vi "Get Random Monitor Edge Point.vi"(7 "Edge":enum16{"Left", "Top", "Right", "Bottom"}(ring), 10 "Monitor Bounds":T2) -> (2 "Point":T1)   [LabVIEW 2019, in "Window.lvlib"]
doc: "Get a random point on the specified edge of a given bounds rectangle, where the point is in the middle 80% of the edge."
uses:
  Window.lvlib
  <vilib>/numeric/Random Number (Range) I64.vi
  _2D/Point.ctl
  _2D/2D.lvlib
  <vilib>/Utility/miscctls.llb/LVRectTypeDef.ctl
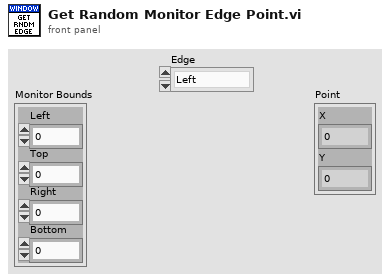
[diagram p1: front panel]
types:
  T1 = typedef "2D.lvlib/Point.ctl" = cluster{"X":i16, "Y":i16}
  T2 = typedef "LVRectTypeDef.ctl" = cluster{"Left":i16, "Top":i16, "Right":i16, "Bottom":i16}
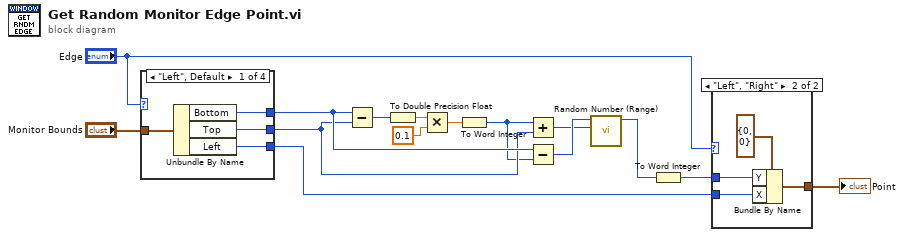
[diagram p0: block diagram]
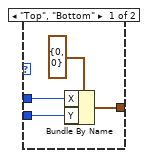
[diagram p2: hidden frame]
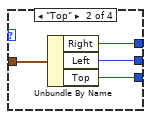
[diagram p3: hidden frame]
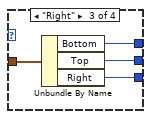
[diagram p4: hidden frame]
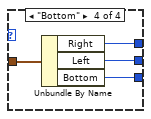
[diagram p5: hidden frame]
diagram:
  n1 = case shown="\"Left\", Default" "Edge" {
    tunnel: [w19 w23 w27 w31] -> w12
    tunnel: [w18 w22 w26 w30] -> w10
    tunnel: "Monitor Bounds" -> [w17 w21 w25 w29]
    tunnel: [w16 w20 w24 w28] -> w6
    frame "Left", Default {
      n2 = Unbundle By Name(w17) -> ("Bottom"=w19:i16, "Top"=w18:i16, "Left"=w16:i16)
    }
    frame "Top" {
      n3 = Unbundle By Name(w21) -> ("Right"=w23:i16, "Left"=w22:i16, "Top"=w20:i16)
    }
    frame "Right" {
      n4 = Unbundle By Name(w25) -> ("Bottom"=w27:i16, "Top"=w26:i16, "Right"=w24:i16)
    }
    frame "Bottom" {
      n5 = Unbundle By Name(w29) -> ("Right"=w31:i16, "Left"=w30:i16, "Bottom"=w28:i16)
    }
  }
  n6 = Subtract(x=w12, y=w10) -> (x-y=w15:i16)
  n7 = To Double Precision Float(number=w15) -> (double precision float=w14:dbl)
  n8 = Multiply(x=w14, y=0.1) -> (x*y=w11:dbl)
  n9 = To Word Integer(number=w11) -> (16bit integer=w5:i16)
  n10 = Add(x=w5, y=w10) -> (x+y=w8:i16)
  n11 = Subtract(x=w12, y=w5) -> (x-y=w9:i16)
  n12 = call-poly <vilib>:"Random Number (Range).vi"("lower bound (-100)"=w8, "upper bound (100)"=w9) -> ("number"=w4:i64)  [unwired: 9 in]
  n13 = To Word Integer(number=w4) -> (16bit integer=w3:i16)
  n14 = case shown="\"Left\", \"Right\"" "Edge" {
    tunnel: w6 -> [w34 w38]
    tunnel: w3 -> [w33 w37]
    tunnel: [w32 w36] -> w2
    frame "Top", "Bottom" {
      n15 = Bundle By Name(cluster=T1 {"X"=0, "Y"=0} ("Position"), "X"=w33, "Y"=w34) -> (w32:T1)
    }
    frame "Left", "Right" {
      n16 = Bundle By Name(cluster=T1 {"X"=0, "Y"=0} ("Position"), "Y"=w37, "X"=w38) -> (w36:T1)
    }
  }
  "Point" <- w2
